vi "close.vi"(8 "error in (no error)":errorcluster, 11 "Torque Transducer in":refnum<class "Torque Transducer.lvclass">) -> (0 "error out":errorcluster, 3 "Torque Transducer out":refnum<class "Torque Transducer.lvclass">)   [LabVIEW 2025, in "Torque Transducer.lvclass"]
uses:
  Torque Transducer.lvclass
  Torque Transducer.lvclass/Torque Transducer.ctl
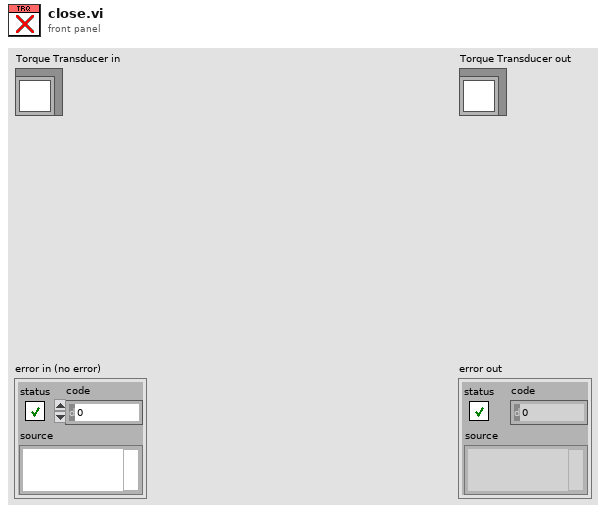
[diagram p1: front panel]
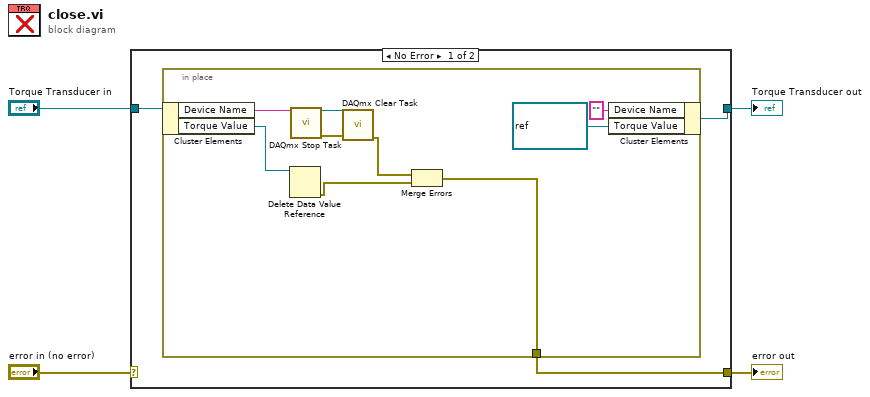
[diagram p0: block diagram]
diagram:
  n1 = case shown="No Error" "error in (no error)" {
    selector: "error in (no error)" -> [_ w18]
    tunnel: [w5 w18] -> w3
    tunnel: [w6 w17] -> w1
    tunnel: "Torque Transducer in" -> [w7 w17]
    frame No Error {
      n2 = in-place {
        in-place-border: [w10] -> w5
        n3 = in-place-cluster #1(w7) -> ("Device Name"=w16:string, "Torque Value"=w8:refnum<data-value>)
        n4 = Delete Data Value Reference(data value reference=w8) -> (error out=w11:errorcluster)  [unwired: 1 in, 1 out]
        n5 = call <vilib>:"DAQmx Stop Task.vi"("task/channels in"=w16) -> ("task out"=w15:refnum<k21>, "error out"=w14:errorcluster)  [unwired: 13 in]
        n6 = call <vilib>:"DAQmx Clear Task.vi"("task in"=w15, "error in"=w14) -> ("error out"=w12:errorcluster)  [unwired: 13 in]
        n7 = Merge Errors(w12, w11) -> (w10:errorcluster)
        n8 = in-place-cluster #1("Device Name"="", "Torque Value"=refnum<data-value> refnum) -> (w6:refnum<class "Torque Transducer.lvclass">)
      }
    }
    frame Error {
    }
  }
  "error out" <- w3
  "Torque Transducer out" <- w1
